vi "Instrument Update.vi"(8 "error in (no error)":errorcluster, 10 "Instrument Record":T1, 11 "Connection Refnum":T2) -> (0 "error out":errorcluster, 2 "Updated Instrument":T1, 3 "Connection Refnum":T2)   [LabVIEW 2011]
uses:
  Instrument Record.ctl
  Summitek EXT/ODBC/SQL Controls/Connection Refnum.ctl
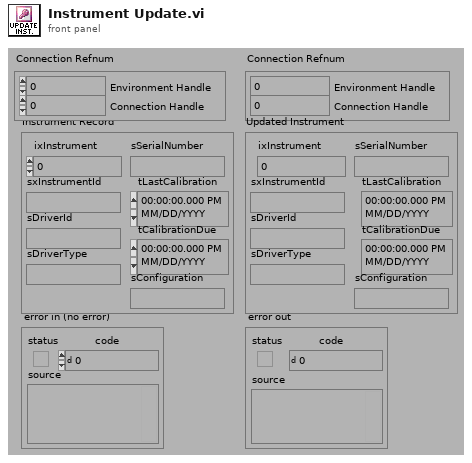
[diagram p1: front panel]
types:
  T1 = typedef "Instrument Record.ctl" = cluster{"ixInstrument":i32, "sxInstrumentId":string, "sDriverId":string, "sDriverType":string, "sSerialNumber":string, "tLastCalibration":timestamp, "tCalibrationDue":timestamp, "sConfiguration":string}
  T2 = typedef "Connection Refnum.ctl" = cluster{"Environment Handle":i32, "Connection Handle":i32}
  T3 = typedef "Statement Refnum.ctl" = cluster{"Statement Handle":i32, "Parameter Number":u16}
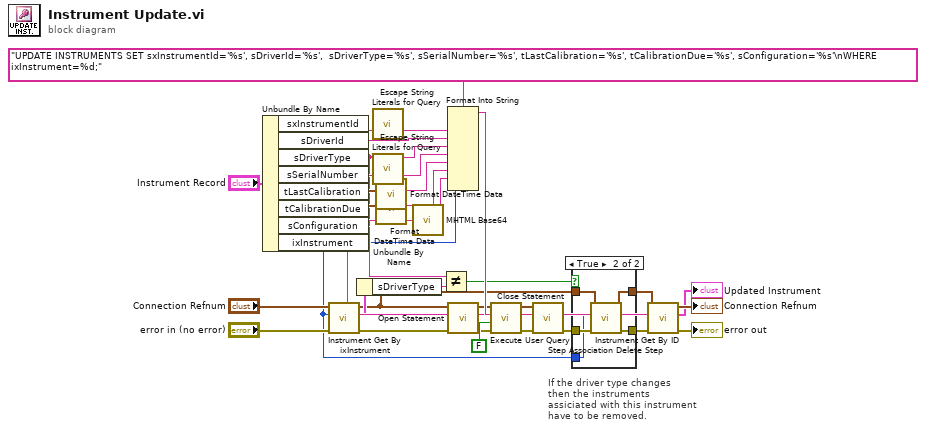
[diagram p0: block diagram]
diagram:
  # "If the driver type changes\nthen the instruments\nassiciated with this instrument\nhave to be removed."
  n1 = Unbundle By Name("Instrument Record") -> ("sxInstrumentId"=w13:string, "sDriverId"=w23:string, "sDriverType"=w3:string, "sSerialNumber"=w15:string, "tLastCalibration"=w18:timestamp, "tCalibrationDue"=w20:timestamp, "sConfiguration"=w26:string, "ixInstrument"=w1:i32)
  n2 = call "Instrument Get By ixInstrument.vi"("error in (no error)"="error in (no error)", "ixInstrument"=w1, "Connection Refnum"="Connection Refnum") -> ("error out"=w10:errorcluster, "Instrument Record"=w9:T1, "Connection Refnum"=w7:T2)  [unwired: 5 in, 1 out]
  n3 = Unbundle By Name(w9) -> ("sDriverType"=w4:string)
  n4 = call "Escape String Literals for Query.vi"("String"=w13) -> ("escaped String"=w16:string)  [unwired: 1 in, 13 out]
  n5 = call "Escape String Literals for Query.vi"("String"=w15) -> ("escaped String"=w14:string)  [unwired: 1 in, 13 out]
  n6 = call "Format DateTime Data.vi"("Timestamp in"=w18) -> ("UTC DB String out"=w17:string)  [unwired: 10 out]
  n7 = call "Format DateTime Data.vi"("Timestamp in"=w20) -> ("UTC DB String out"=w19:string)  [unwired: 10 out]
  n8 = call "MHTML Base64.vi"("Binary String"=w26) -> ("String (Base64)"=w25:string)  [unwired: 14 out]
  n9 = Not Equal?(x=w3, y=w4) -> (x != y?=w2:bool)
  n10 = Format Into String(format string="UPDATE INSTRUMENTS SET sxInstrumentId='%s', sDriverId='%s',  sDriverType='%s', sSerialNumber='%s', tLastCalibration='%s', tCalibrationDue='%s', sConfiguration='%s'\nWHERE ixInstrument=%d;" ("User Query"), w16, w23, w3, w14, w17, w19, w25, w1) -> (resulting string=w29:string)  [unwired: 2 in, 1 out]
  n11 = call "Open Statement.vi"("error in (no error)"=w10, "Connection Refnum"=w7) -> ("error out"=w28:errorcluster, "Statement Refnum"=w27:T3)  [unwired: 4 out]
  n12 = call "Execute User Query.vi"("error in (no error)"=w28, "Return Data? (f)"=FALSE, "User Query"=w29, "Statement Refnum"=w27) -> ("error out"=w32:errorcluster, "Statement Refnum"=w31:T3)  [unwired: 2 out]
  n13 = call "Close Statement.vi"("error in (no error)"=w32, "Statement Refnum"=w31) -> ("error out"=w8:errorcluster)  [unwired: 5 out]
  n14 = case shown="True" w2 {
    tunnel: w7 -> [w36 w38]
    tunnel: w8 -> [w35 w41]
    tunnel: [w36 w39] -> w6
    tunnel: [w35 w40] -> w5
    tunnel: w1 -> [_ w37]
    frame False {
    }
    frame True {
      n15 = call "Step Association Delete Step.vi"("error in (no error)"=w41, "iStep (0)"=w37, "Connection Refnum"=w38) -> ("error out"=w40:errorcluster, "Connection Refnum"=w39:T2)  [unwired: 7 in]
    }
  }
  n16 = call "Instrument Get By ID.vi"("error in (no error)"=w5, "sxInstrumentId (\"\")"=w13, "Connection Refnum"=w6) -> ("error out"=→"error out":errorcluster, "Instrument Record"=→"Updated Instrument":T1, "Connection Refnum"=→"Connection Refnum":T2)  [unwired: 6 out]
